vi "Get All Channels.vi"(8 "error in (no error)":errorcluster, 10 "Default Channel Status":bool, 11 "Module Configuration":refnum<class "Module Configuration.lvclass">=refnum) -> (0 "error out":errorcluster, 1 "Output Channels[]":refnum<class "Output Channels.lvclass">[](array[class]), 2 "Input Channels[]":refnum<class "Input Channels.lvclass">[](array[class]), 3 "Module Configuration out":refnum<class "Module Configuration.lvclass">, 4 "All Active Channels[]":T1[](array[typedef]))   [LabVIEW 2020, in "Plugin.lvlib" / "Plugin_UI.lvclass"]
doc: "This VI initiates the clusters disable, weight config and ChannelInfo by reading from file or sets defualt value if new plugin is loaded."
uses:
  Plugin_UI.lvclass
  builds/Libraries/LabSys Framework.lvlibp/Configuration Storage/Module Configuration/Module Configuration.lvclass
  Channels/Input Channels/Input Channels.lvclass
  Channels/Output Channels/Output Channels.lvclass
  builds/Libraries/LabSys Framework.lvlibp/Configuration Storage/Test Configuration/Channel Information.ctl
  builds/Libraries/LabSys Framework.lvlibp/Configuration Storage/Test Configuration/Channel Directions.ctl
  builds/Libraries/LabSys Framework.lvlibp/Configuration Storage/Test Configuration/Scaling Information.ctl
  builds/Libraries/LabSys Framework.lvlibp/Configuration Storage/Test Configuration/Scaling Types.ctl
  builds/Libraries/Framework Base Library.lvlibp/Value Types.ctl
  builds/Libraries/LabSys Framework.lvlibp/Configuration Storage/Test Configuration/Subchannel Information.ctl
  Auxiliary Data.ctl
  Channels/Plugin_Channels.lvclass
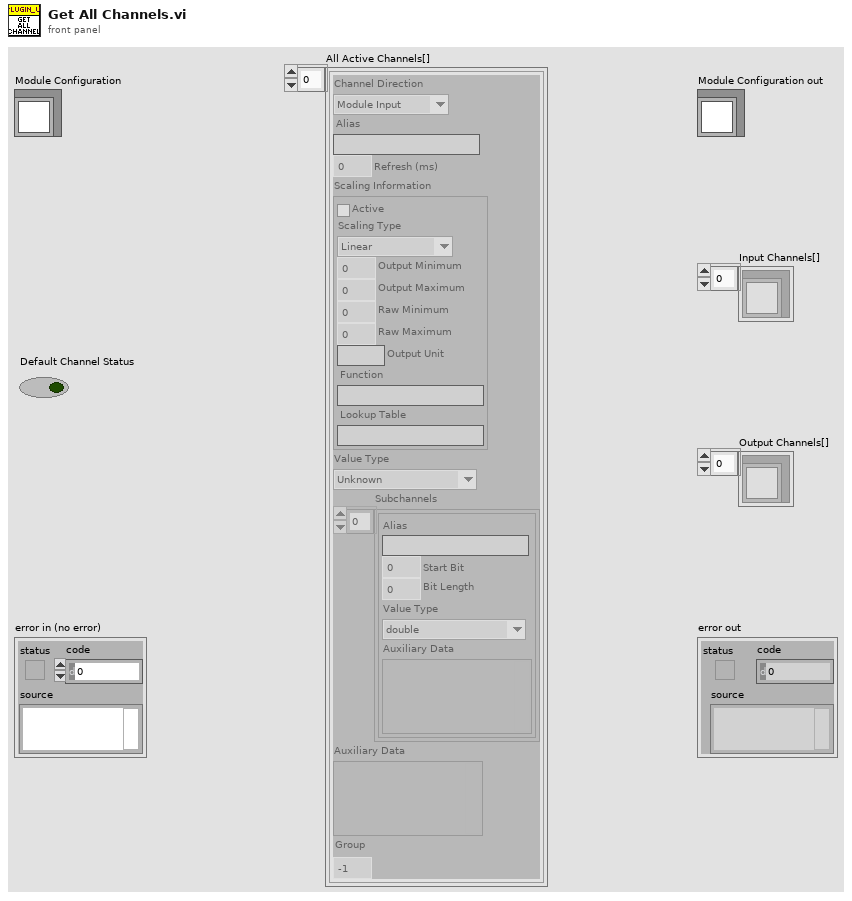
[diagram p1: front panel]
types:
  T1 = typedef "LabSys Framework.lvlibp/Configuration Storage.lvlib/Test Configuration.lvclass/Channel Information.ctl" = cluster{"Channel Direction":T2, "Alias":string, "Refresh (ms)":dbl, "Scaling Information":T3, "Value Type":T5, "Subchannels":T6[], "Auxiliary Data":variant, "Group":i32}
  T2 = typedef "LabSys Framework.lvlibp/Configuration Storage.lvlib/Test Configuration.lvclass/Channel Directions.ctl" = enum8{"Module Input", "Module Output"}
  T3 = typedef "LabSys Framework.lvlibp/Configuration Storage.lvlib/Test Configuration.lvclass/Scaling Information.ctl" = cluster{"Active":bool, "Scaling Type":T4, "Output Minimum":dbl, "Output Maximum":dbl, "Raw Minimum":dbl, "Raw Maximum":dbl, "Output Unit":string, "Function":string, "Lookup Table":string}
  T4 = typedef "LabSys Framework.lvlibp/Configuration Storage.lvlib/Test Configuration.lvclass/Scaling Types.ctl" = enum8{"Linear", "Function", "Lookup Table"}
  T5 = typedef "Framework Base Library.lvlibp/Value Types.ctl" = enum8{"Unknown", "double", "double array", "Waveform", "DigWaveform", "Boolean", "Decimal", "String", "Db2Message", "Byte Array", "Unsigned Decimal"}
  T6 = typedef "LabSys Framework.lvlibp/Configuration Storage.lvlib/Test Configuration.lvclass/Subchannel Information.ctl" = cluster{"Alias":string, "Start Bit":u32, "Bit Length":u32, "Value Type":T5, "Auxiliary Data":variant}
  T7 = typedef "Plugin.lvlib/Plugin_UI.lvclass/Auxiliary Data.ctl" = cluster{"Plugin_Data":refnum<class "Plugin_Channels.lvclass">}
  T8 = typedef "Plugin.lvlib/Plugin_Channels.lvclass/Channel Type.ctl" = enum16{"Input", "Output"}
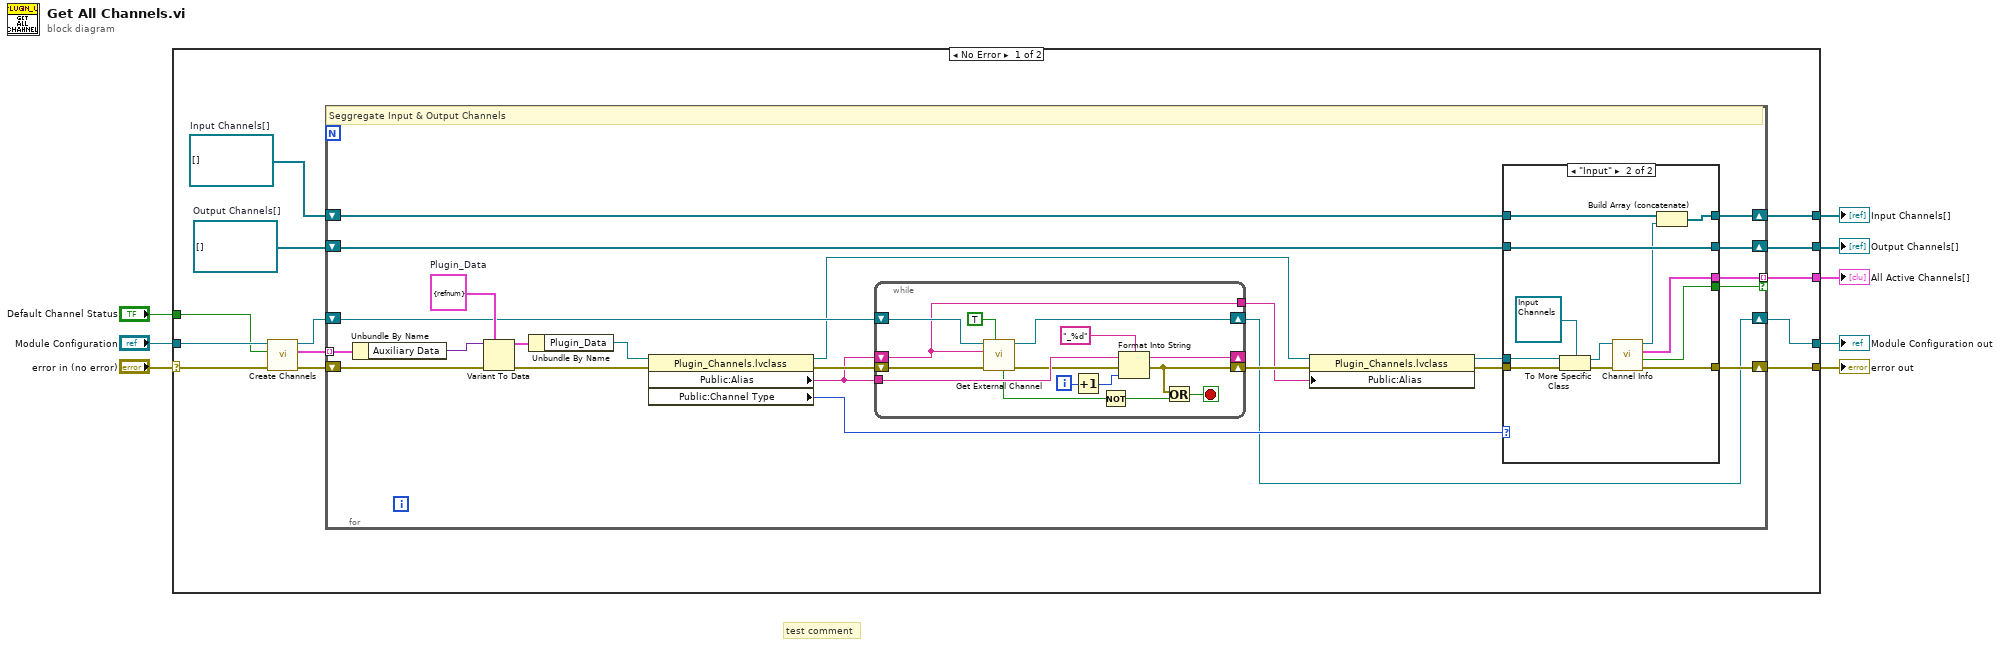
[diagram p0: block diagram]
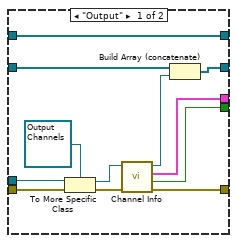
[diagram p2: hidden frame]
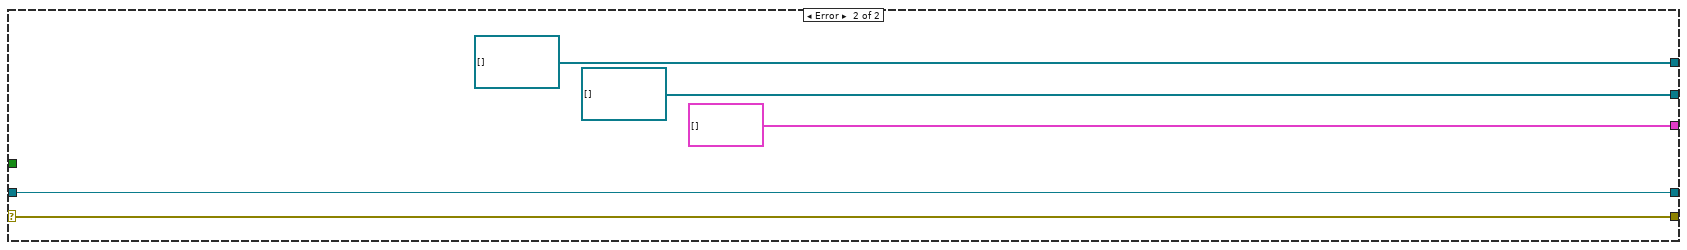
[diagram p3: hidden frame]
diagram:
  # "test comment"
  n1 = case shown="No Error" "error in (no error)" {
    selector: "error in (no error)" -> [w16 w89]
    tunnel: [w21 w89] -> w8
    tunnel: [w20 w88] -> w7
    tunnel: "Module Configuration" -> [w17 w88]
    tunnel: "Default Channel Status" -> [w12 _]
    tunnel: [w19 refnum<class "Input Channels.lvclass">[] [] ("Input Channels[]")] -> w5
    tunnel: [w18 refnum<class "Output Channels.lvclass">[] [] ("Output Channels[]")] -> w4
    tunnel: [w11 T1[] []] -> w1
    frame No Error {
      w9 = refnum<class "Input Channels.lvclass">[] []  # Input Channels[]
      w10 = refnum<class "Output Channels.lvclass">[] []  # Output Channels[]
      n2 = call "Create Channels.vi"("error in (no error)"=w16, "Default Channel Status"=w12, "Module Configuration in"=w17) -> ("error out"=w15:errorcluster, "All Channels[]"=w13:T1[], "Module Configuration out"=w14:refnum<class "Module Configuration.lvclass">)  [unwired: 6 in]
      n3 = for {
        shift-right: [w41] -> w21
        shift-left: w15 -> [w43]
        tunnel: w13 -> [w45] mode=indexing
        shift-right: [w40] -> w18
        shift-left: w10 -> [w39]
        shift-right: [w38] -> w19
        shift-left: w9 -> [w37]
        shift-right: [w25] -> w20
        shift-left: w14 -> [w32]
        tunnel: [w24] -> w11 mode=indexing if=w22
        w36 = T7 {"Plugin_Data"=refnum}  # Plugin_Data
        # "Seggregate Input & Output Channels"
        n4 = Unbundle By Name(w45) -> ("Auxiliary Data"=w44:variant)
        n5 = Variant To Data(error in=w43, type=w36, Variant=w44) -> (data=w35:T7, error out=w42:errorcluster)
        n6 = Unbundle By Name(w35) -> ("Plugin_Data"=w34:refnum<class "Plugin_Channels.lvclass">)
        n7 = property class="Plugin_Channels.lvclass"(reference=w34, error in=w42) -> (reference out=w27:refnum<class "Plugin_Channels.lvclass">, error out=w33:errorcluster, "Public:Alias"=w30:string, "Public:Channel Type"=w31:T8)
        n8 = while {
          shift-right: [w55] -> w29
          shift-left: w33 -> [w52]
          shift-right: [w60] -> _
          shift-left: w30 -> [w46]
          tunnel: w30 -> [w59]
          shift-right: [w49] -> w25
          shift-left: w32 -> [w50]
          tunnel: [w46] -> w23
          i -> [w58]
          stop <- w54 stop-if-true
          n9 = call "Get External Channel.vi"("Ignore Module Channels (F)"=TRUE, "error in (no error)"=w52, "Channel Name"=w46, "Module Configuration in"=w50) -> ("error out"=w51:errorcluster, "Module Configuration out"=w49:refnum<class "Module Configuration.lvclass">, "Channel Configuration Found"=w47:bool)  [unwired: 3 in, 2 out]
          n10 = Increment(x=w58) -> (x+1=w53:i32)
          n11 = Not(x=w47) -> (.not. x?=w56:bool)
          n12 = Format Into String(format string="_%d", initial string=w59, error in=w51, w53) -> (resulting string=w60:string, error out=w55:errorcluster)
          n13 = Or(x=w55, y=w56) -> (x .or. y?=w54:bool)
        }
        n14 = property class="Plugin_Channels.lvclass"(reference=w27, error in=w29, "Public:Alias"=w23) -> (reference out=w26:refnum<class "Plugin_Channels.lvclass">, error out=w28:errorcluster)
        n15 = case shown="\"Input\"" w31 {
          tunnel: w28 -> [w72 w84]
          tunnel: w26 -> [w71 w83]
          tunnel: [w65 w78] -> w41
          tunnel: [w69 w82] -> w40
          tunnel: w39 -> [w68 w82]
          tunnel: [w67 w81] -> w38
          tunnel: w37 -> [w67 w80]
          tunnel: [w62 w75] -> w24
          tunnel: [w61 w74] -> w22
          frame "Output" {
            n16 = To More Specific Class(target class=refnum<class "Output Channels.lvclass"> refnum ("Plugin.lvlib:Output Channels.lvclass"), reference=w71, error in=w72) -> (specific class reference=w64:refnum<class "Output Channels.lvclass">, error out=w66:errorcluster)
            n17 = call-dynamic "Channel Info.vi"("error in"=w66, "Output Channels in"=w64) -> ("error out"=w65:errorcluster, "Channel Active?"=w61:bool, "Channel Information"=w62:T1, "Output Channels out"=w63:refnum<class "Output Channels.lvclass">)  [unwired: 6 in]
            n18 = Build Array (concatenate)(w68, w63) -> (w69:refnum<class "Output Channels.lvclass">[])
          }
          frame "Input" {
            n19 = To More Specific Class(target class=refnum<class "Input Channels.lvclass"> refnum ("Plugin.lvlib:Input Channels.lvclass"), reference=w83, error in=w84) -> (specific class reference=w77:refnum<class "Input Channels.lvclass">, error out=w79:errorcluster)
            n20 = call-dynamic "Channel Info.vi"("error in"=w79, "Input Channels in"=w77) -> ("error out"=w78:errorcluster, "Channel Active?"=w74:bool, "Channel Information"=w75:T1, "Input Channels out"=w76:refnum<class "Input Channels.lvclass">)  [unwired: 6 in]
            n21 = Build Array (concatenate)(w80, w76) -> (w81:refnum<class "Input Channels.lvclass">[])
          }
        }
      }
    }
    frame Error {
    }
  }
  "error out" <- w8
  "Module Configuration out" <- w7
  "Input Channels[]" <- w5
  "Output Channels[]" <- w4
  "All Active Channels[]" <- w1
